vi "Module - Page Master Data.vi"(11 "Stop":bool) -> ()   [LabVIEW 2020]
uses:
  Control/Setup - Sequence Data.ctl
  Control/State - eFGV.ctl
panel:
  in  "Tab Control":enum32{"Test Procedure", "Layout"}(tab)
  in  "Header multi-test":T1={"Test Type"="Test Requirement", "Seq.Done"="Done", "Seq.No"="No.", "Seq.SelectRun"="Run", "Seq.SelectRun 2"="Test Sequence", "Seq.SelectRun 3"="Test Requirement ID", "Test Type 2"="Test Procedure", "Test Type 3"="psi", "Test Type 4"="Test Pressure", "Test Type 5"="Secondary", "Test Type 6"="Tertiary", "Test Type 7"="Primary", "Test Type 8"="Holding Time (hh:mm)", "Test Type 9"="Section", "Test Type 10"="Test Media", "Test Type 11"="psi", "Test Type 12"="Actuator Pressure", "Test Type 13"="psi/hour", "Test Type 14"="Chart scale", "Test Type 15"="2nd", "Test Type 16"="3rd", "Test Type 17"="1st", "Test Type 18"="Blowdown", "Test Type 19"="psi", "Test Type 20"="Max. Blowdown Pressure", "Seq.SelectRun 4"=""}
  in  "SequenceList":T2[](array[typedef])
  out "Procedure Details Label":string="Procedure Details" caption="Procedure Details"
  out "Indicator.PSL":string caption="PSL"
  out "Indicator.Rev.":string caption="Rev."
  out "Indicator.Procedure No./Ref.":string caption="Procedure No./Ref."
  in  "Procedure Detail.Save":bool
  in  "Button.Edit.Test Procedure.":bool caption="Edit"
  in  "Button.New.Test Procedure":bool caption="New"
  in  "Button.Test Procedure.Copy":bool caption="Copy"
  in  "Button.Search.Test Procedure":bool caption="Search"
  in  "PSL.Control":string(combo) caption="PSL"
  in  "Rev.Control":string caption="Rev."
  in  "Procedure No./Ref.Control":string caption="Procedure No./Ref."
  out "Test Procedure.Selection Label":string="Selection" caption="Selection Label"
  out "Test Procedure Label":string="Test Procedure"
  out "Control.Layout Technical Name":string caption="Layout Technical Name"
  in  "Checkbox.Output":bool caption="Output"
  in  "Checkbox.Default":bool caption="Default"
  in  "Control.Layout Name":string caption="Layout Name"
  in  "Conntrol.Layout ID":u16 caption="Layout ID"
  out "Indicator.Output Name":string caption="Output Name"
  in  "Listbox.Output Type":string(combo) caption="Output Type"
  in  "Control.Company Name":string caption="Company Name"
  out "Indicator.Output Set":u16 caption="Output Set"
  out "Ouput.Layout Detail Label":string="Layout Detail"
  in  "Button.Output.Search":bool caption="Search"
  in  "Button.Edit.Output":bool caption="Edit"
  in  "Button.New.Output":bool caption="New"
  in  "Button.Output.Copy":bool caption="Copy"
  out "Company Name.Indicator":string
  out "Ouput.Selection Label":string="Selection"
  in  "Control.Output Set":u16 caption="Output Set"
  out "Output Label":string="Output"
  # "MASTER DATA"
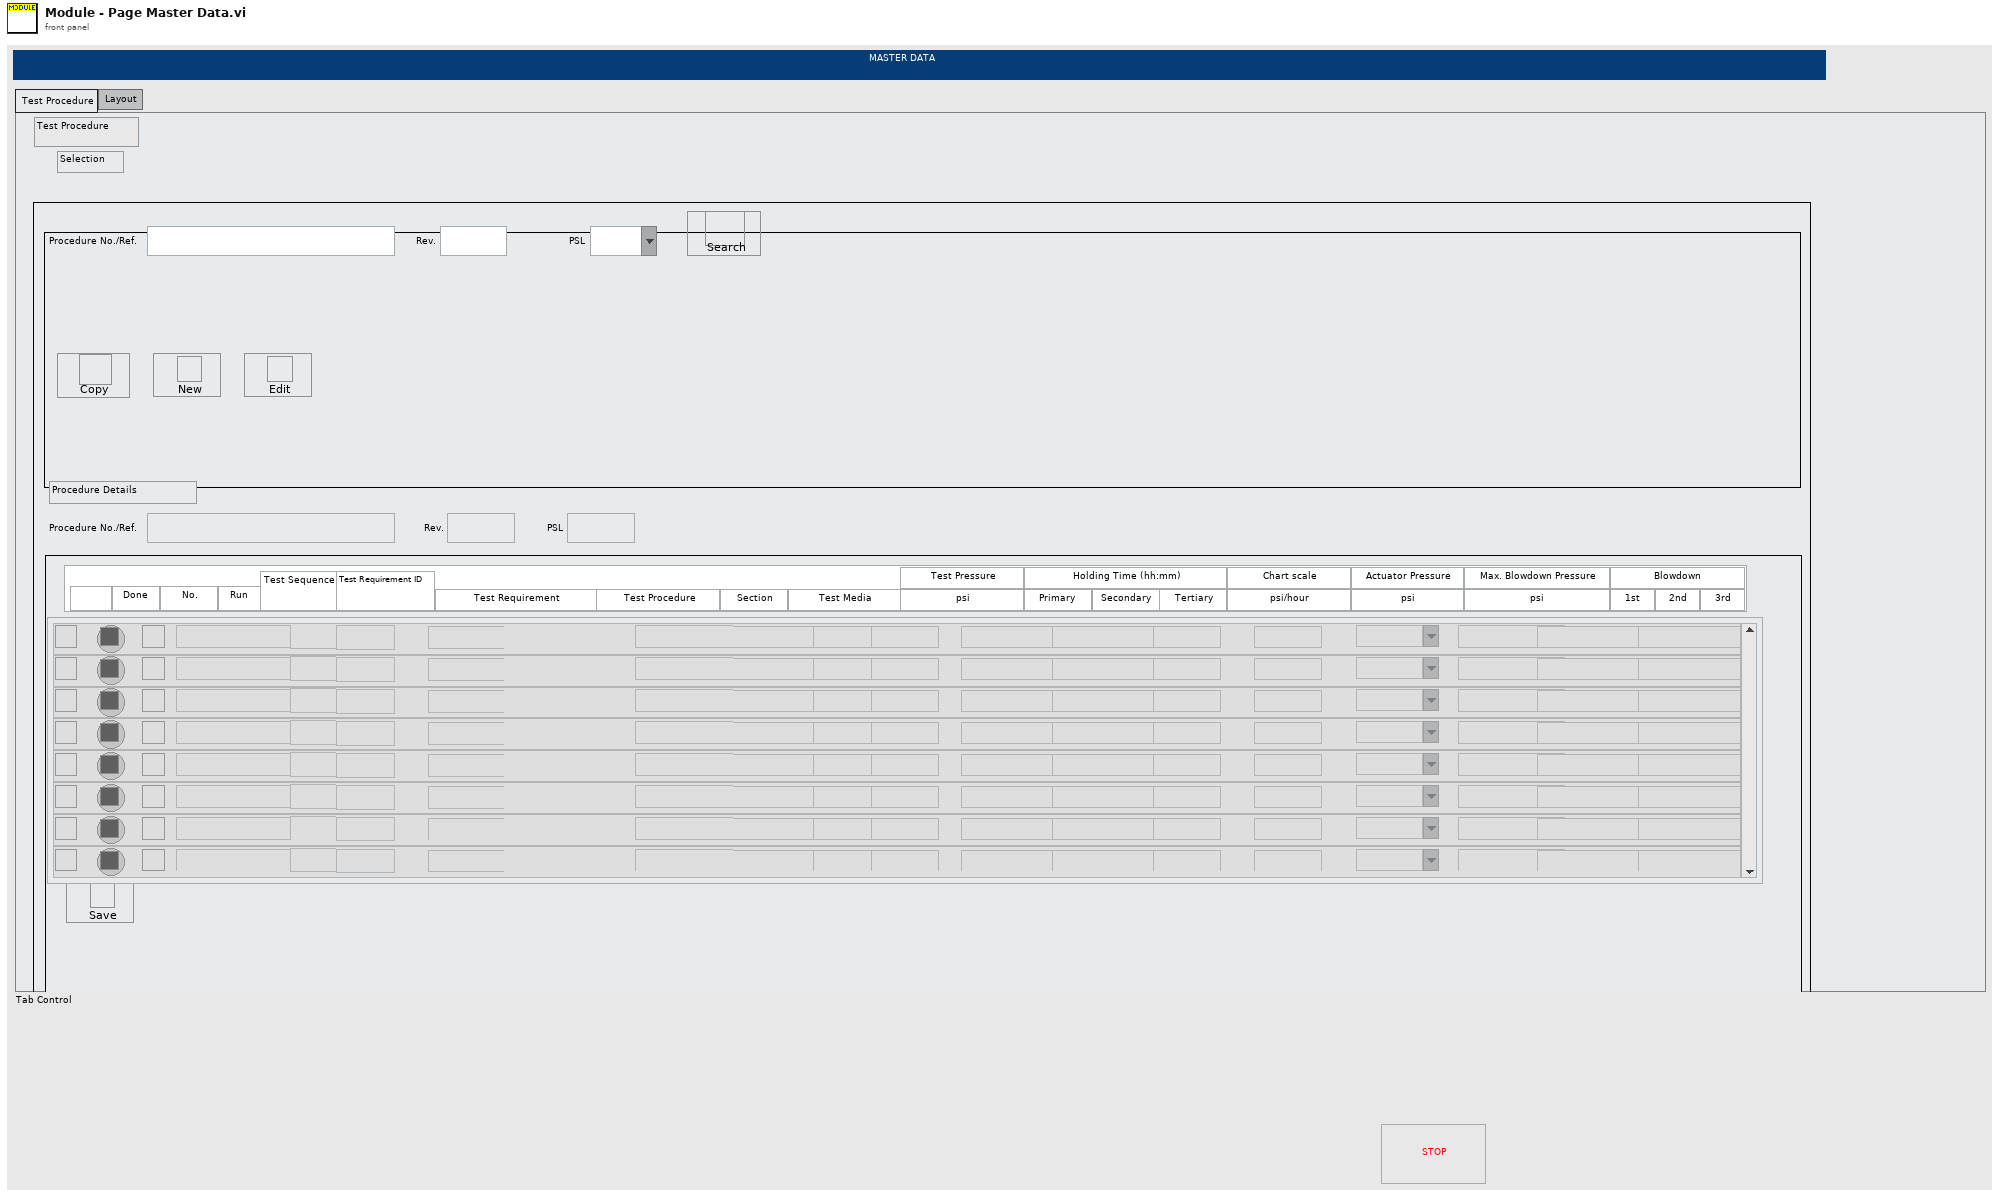
[diagram p1: front panel]
types:
  T1 = cluster{"Test Type":string, "Seq.Done":string, "Seq.No":string, "Seq.SelectRun":string, "Seq.SelectRun 2":string, "Seq.SelectRun 3":string, "Test Type 2":string, "Test Type 3":string, "Test Type 4":string, "Test Type 5":string, "Test Type 6":string, "Test Type 7":string, "Test Type 8":string, "Test Type 9":string, "Test Type 10":string, "Test Type 11":string, "Test Type 12":string, "Test Type 13":string, "Test Type 14":string, "Test Type 15":string, "Test Type 16":string, "Test Type 17":string, "Test Type 18":string, "Test Type 19":string, "Test Type 20":string, "Seq.SelectRun 4":string}
  T2 = typedef "Setup - Sequence Data.ctl" = cluster{"Seq.Select":bool, "Seq.Status":u32, "Seq.Run":bool, "Seq.TestSequence":string, "Seq.No":string, "Seq.ReqID":string, "Seq.TestReq":string, "Seq.Variance":string, "Seq.TestProcedure":string, "Seq.Section":string, "Seq.TestBunker":string, "Seq.TestMedia":string, "Seq.TestPressure":string, "Seq.Cycle":string, "Seq.HoldingTime":string, "Seq.ChartScale":string, "Seq.BDIndicator":string, "Seq.ActuatorPressure":string, "Seq.MaxBDPressure":string}
  T3 = cluster{"T_Out":i32, "Event Ref":refnum<event-registration>}
  T4 = enum16{"Init", "Register Event", "Idle", "Process", "Close"}
  T5 = typedef "State - eFGV.ctl" = enum16{"Init", "Read", "Write", "Exit"}
  T6 = enum32{"invalid app kind", "Development System", "Run Time System", "Student Edition", "Embedded LabVIEW", "Evaluation", "Custom"}
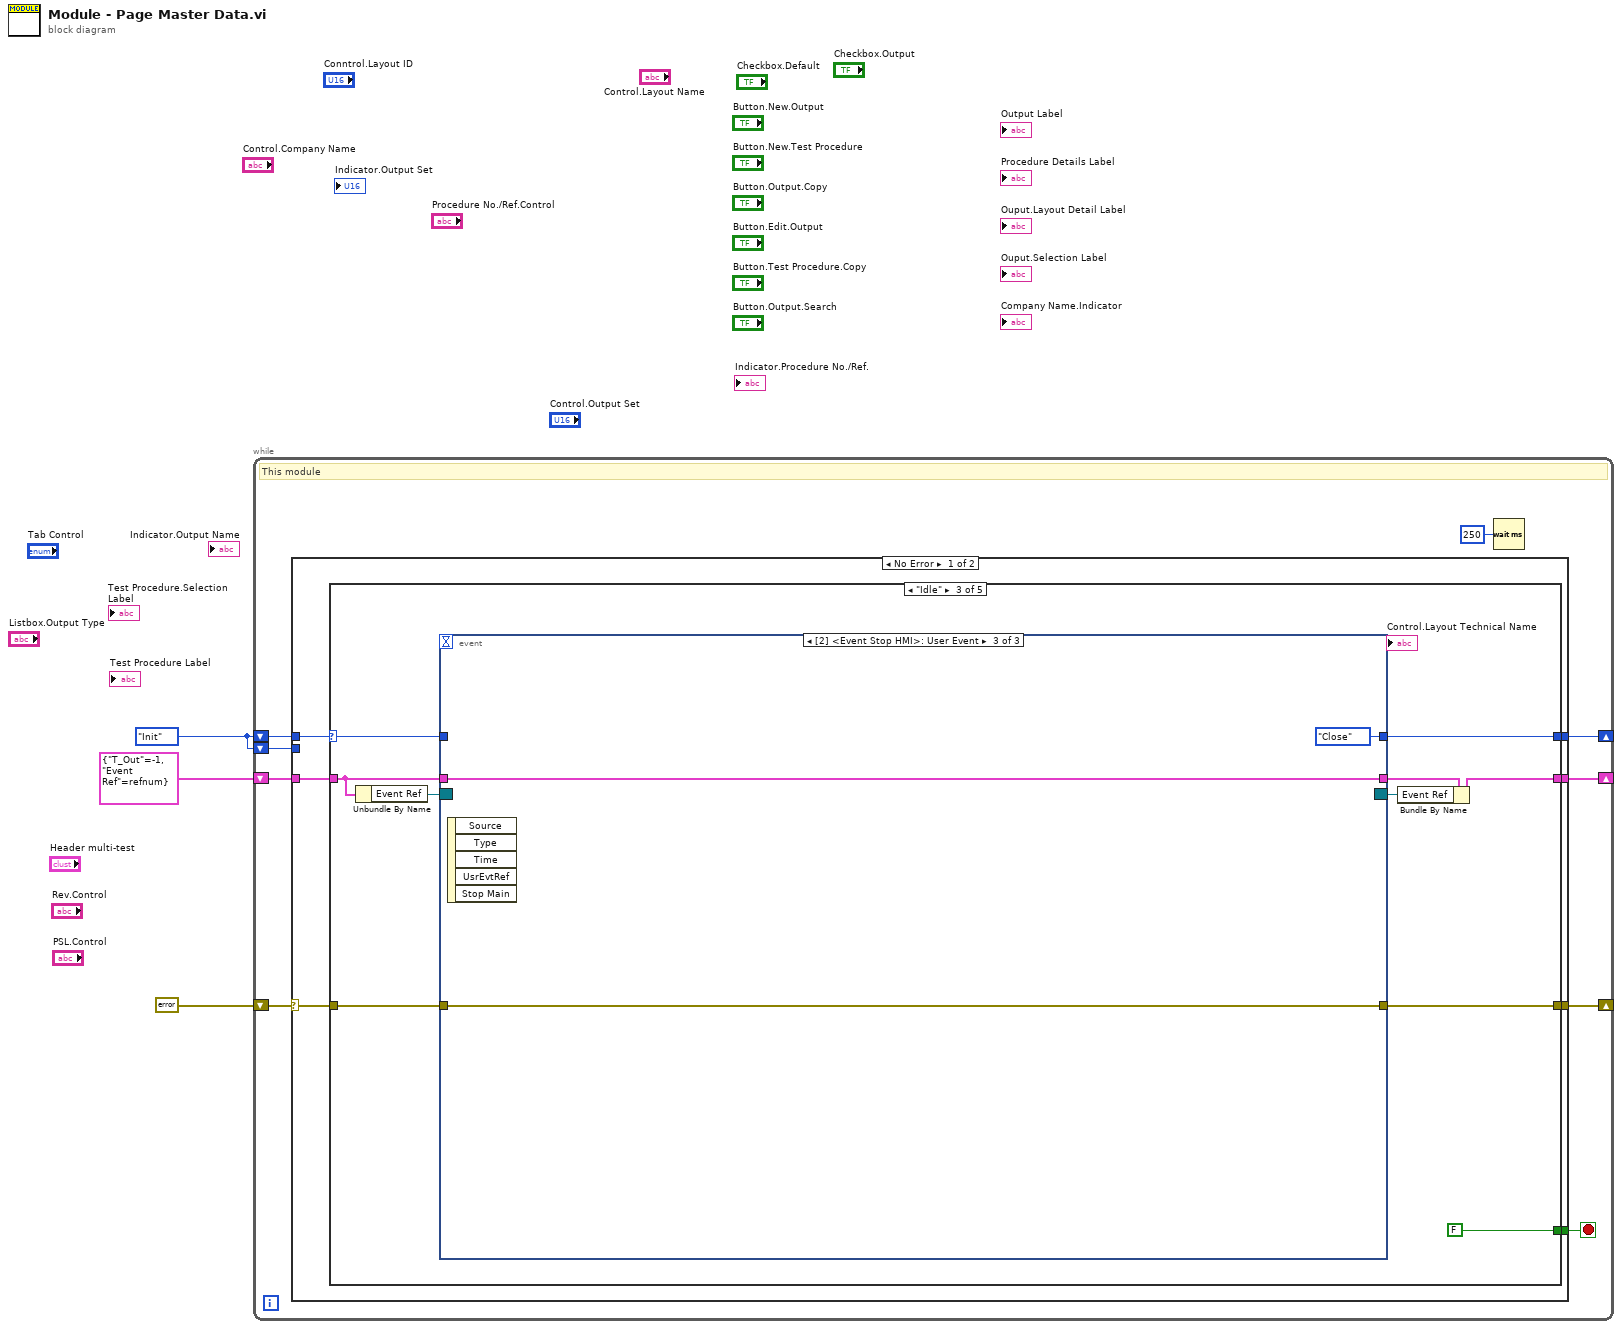
[diagram p0: block diagram]
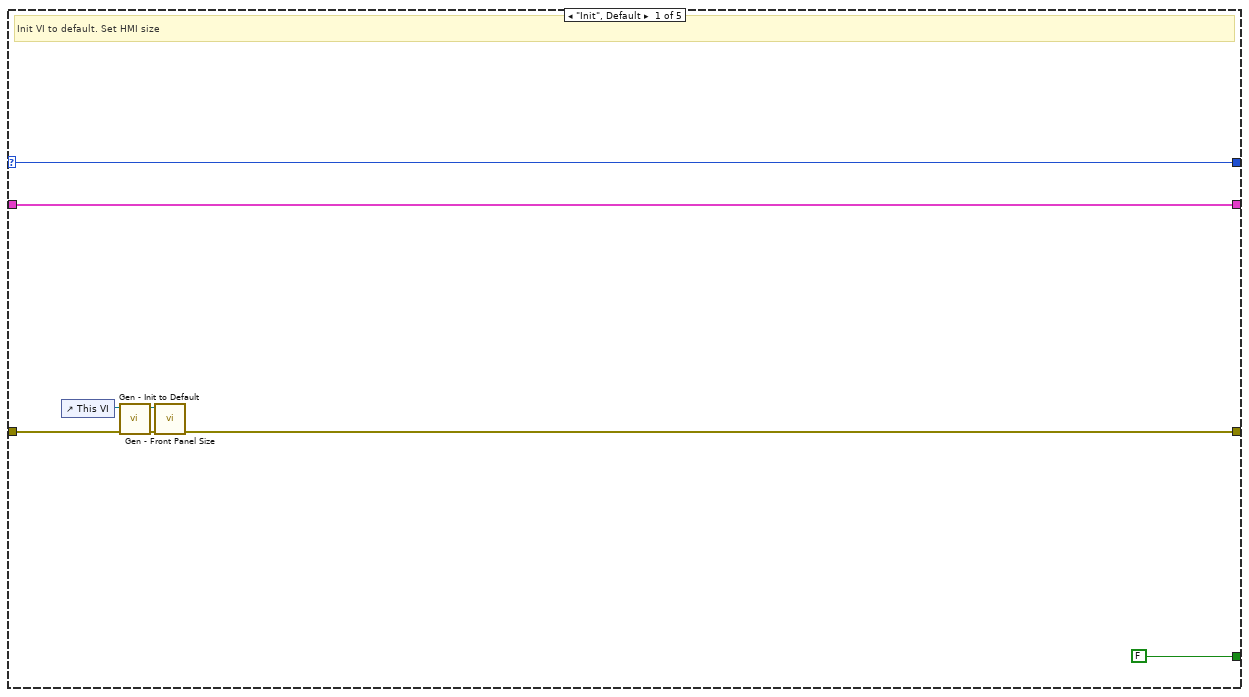
[diagram p2: hidden frame]
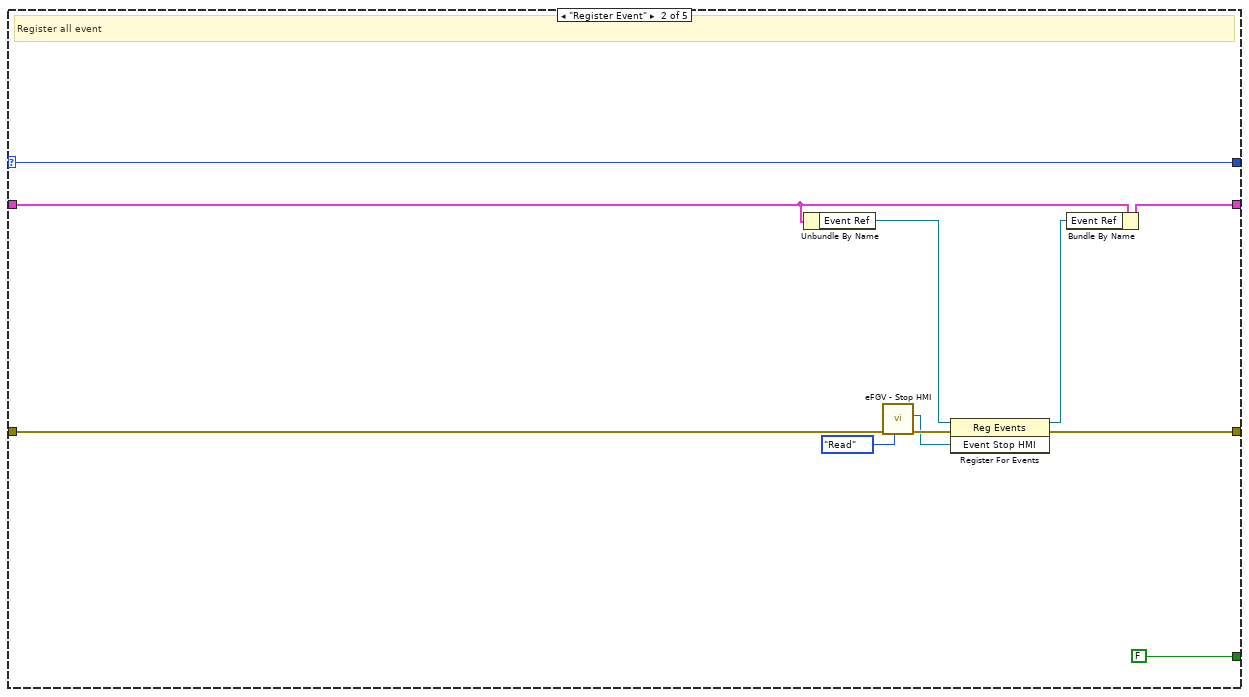
[diagram p3: hidden frame]
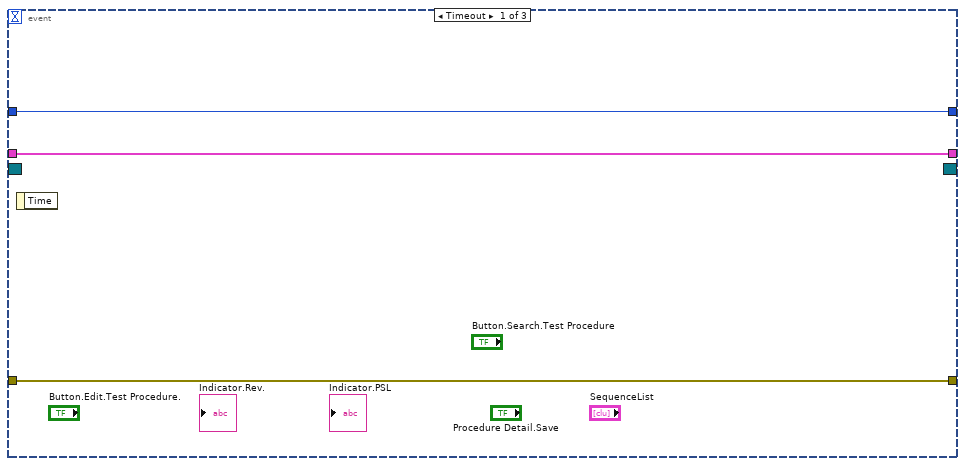
[diagram p4: hidden frame]
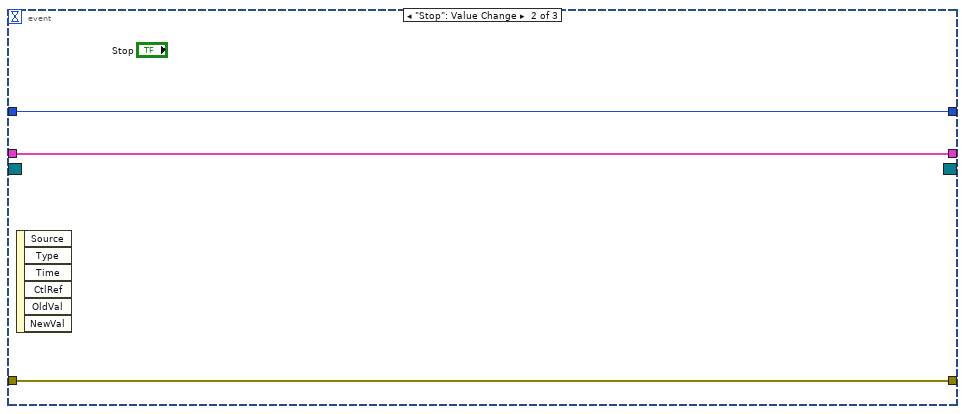
[diagram p5: hidden frame]
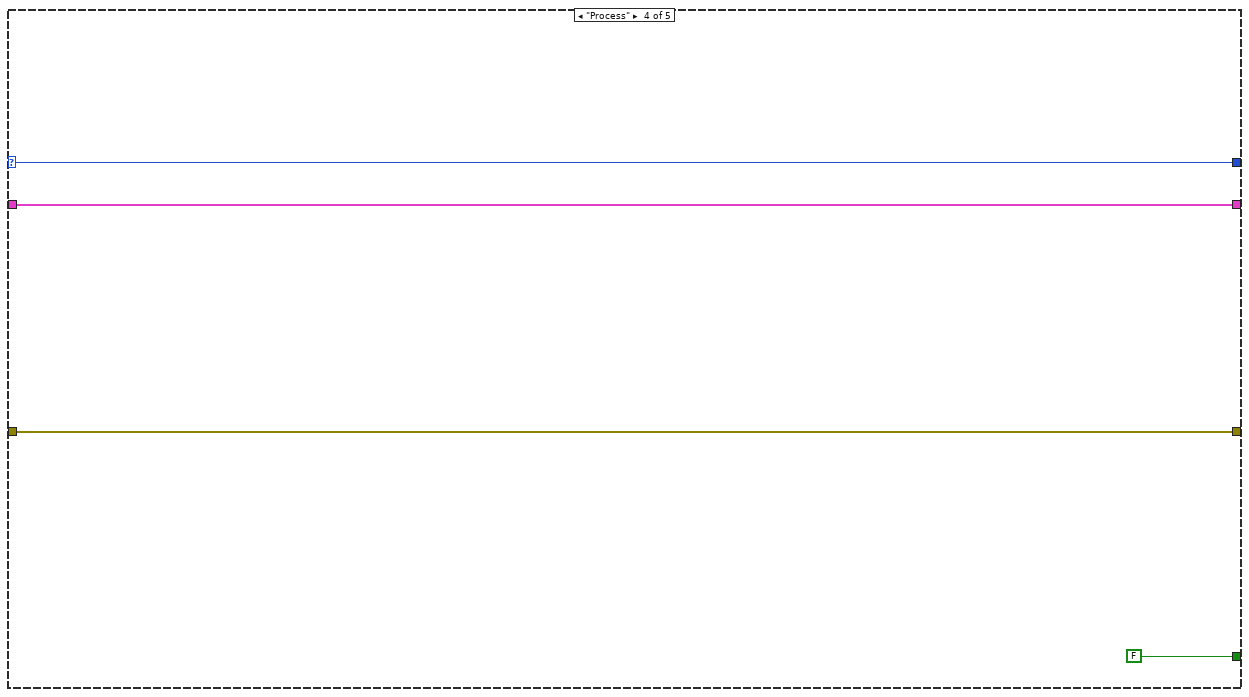
[diagram p6: hidden frame]
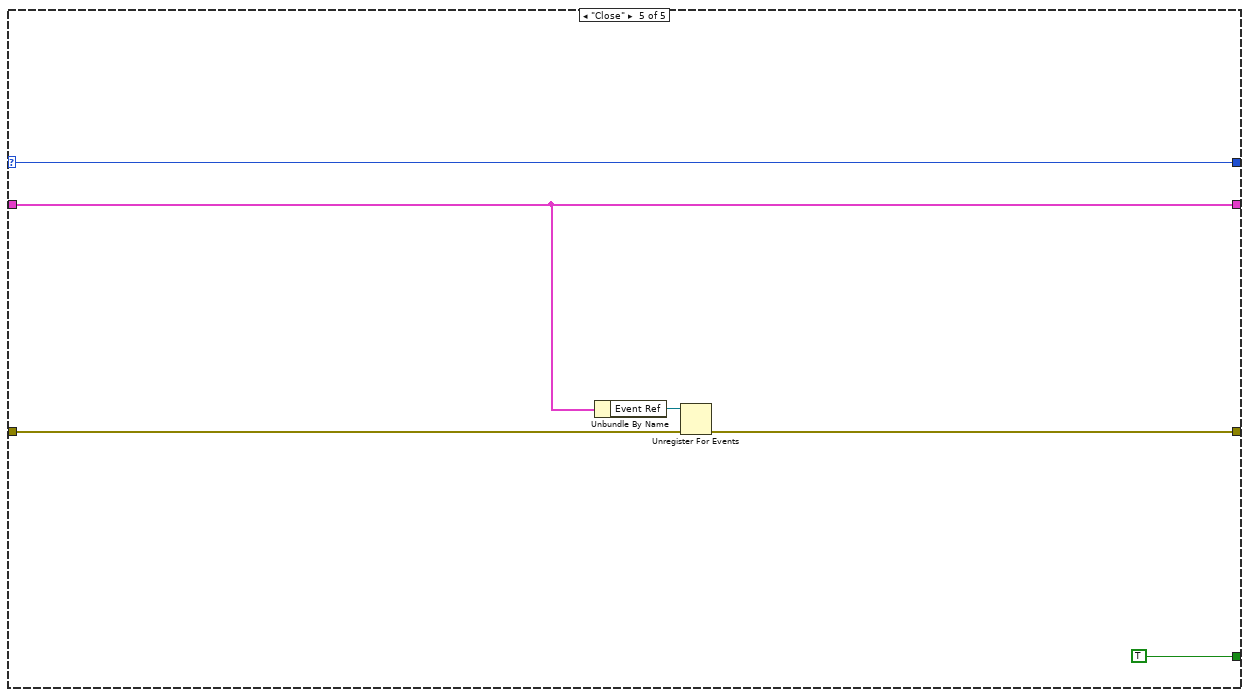
[diagram p7: hidden frame]
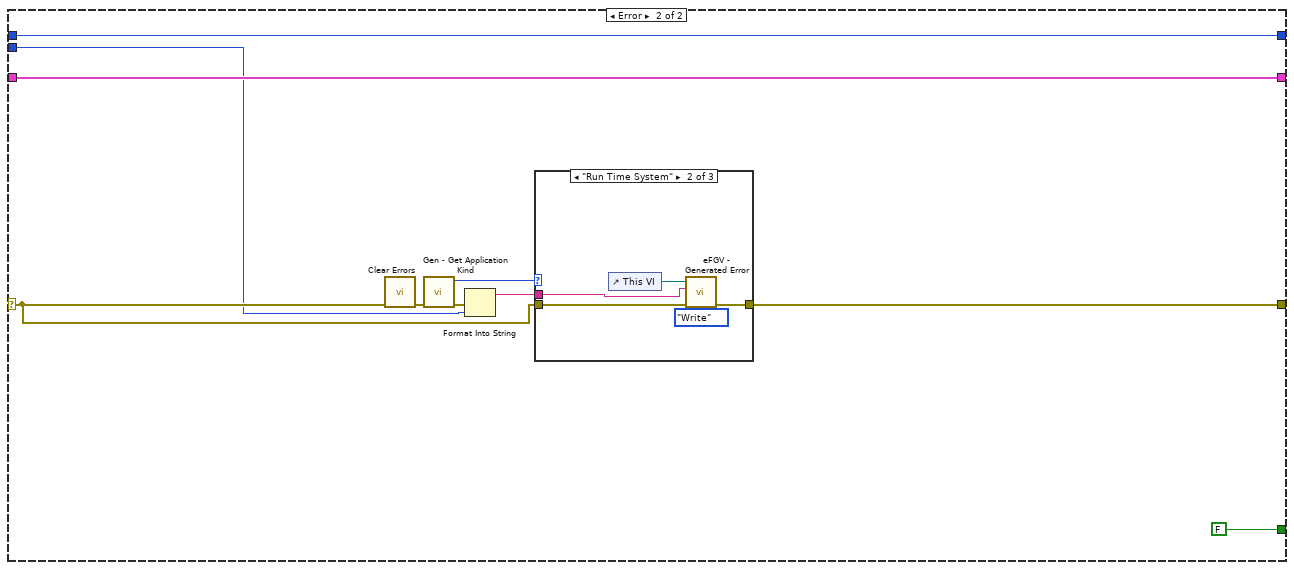
[diagram p8: hidden frame]
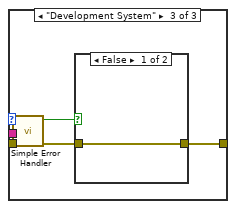
[diagram p10: hidden frame]
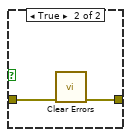
[diagram p11: hidden frame]
diagram:
  w1 = T4."Init"
  n1 = while {
    shift-right: [w8] -> _
    shift-left: w1 -> [w10]
    shift-right: [w11] -> _
    shift-left: errorcluster {"status"=FALSE, "code"=0, "source"=""} ("Error In") -> [w12]
    shift-right: [w6] -> _
    shift-left: T3 {"T_Out"=-1, "Event Ref"=refnum} -> [w7]
    shift-left: w1 -> [w4]
    stop <- w9 stop-if-true
    # "This module"
    n2 = case shown="No Error" w12 {
      selector: w12 -> [w18 w71]
      tunnel: w10 -> [w17 w76]
      tunnel: [w19 w72] -> w11
      tunnel: [w16 FALSE] -> w9
      tunnel: [w15 w76] -> w8
      tunnel: w7 -> [w14 w75]
      tunnel: [w13 w75] -> w6
      tunnel: w4 -> [_ w68]
      frame No Error {
        n3 = case shown="\"Idle\"" w17 {
          selector: w17 -> [w22 w34 w43 w58 w65]
          tunnel: [w25 w38 w48 w61 w66] -> w19
          tunnel: w18 -> [w27 w36 w47 w61 w67]
          tunnel: [FALSE FALSE FALSE FALSE TRUE] -> w16
          tunnel: [w22 w34 w45 w58 w65] -> w15
          tunnel: w14 -> [w24 w31 w42 w59 w63]
          tunnel: [w24 w29 w40 w59 w63] -> w13
          frame "Init", Default {
            # "Init VI to default. Set HMI size"
            n4 = control-ref of="This VI"() -> (w21:refnum<vi>)
            n5 = call "Gen - Init to Default.vi"("Error in"=w27, "This VI"=w21) -> ("Error out"=w26:errorcluster, "This VI Copy"=w20:refnum<vi>)  [unwired: 8 in]
            n6 = call "Gen - Front Panel Size.vi"("Error In"=w26, "This VI"=w20) -> ("Error Out"=w25:errorcluster)  [unwired: 9 in]
          }
          frame "Register Event" {
            # "Register all event"
            n7 = Unbundle By Name(w31) -> ("Event Ref"=w30:refnum<event-registration>)
            n8 = call "eFGV - Stop HMI.vi"("Action"=State_-_eFGV."Read", "Error In"=w36) -> ("Error Out"=w37:errorcluster, "Event Stop HMI"=w33:refnum<user-event>)  [unwired: 7 in, 1 out]
            n9 = register-events(reference=w30, error in=w37, w33) -> (reference out=w28:refnum<event-registration>, error out=w38:errorcluster)
            n10 = Bundle By Name(cluster=w31, "Event Ref"=w28) -> (w29:T3)
          }
          frame "Idle" {
            n11 = Unbundle By Name(w42) -> ("Event Ref"=w41:refnum<event-registration>)
            n12 = event shown="[2] <Event Stop HMI>: User Event" {
              selector: w41 -> [_ _ _]
              dyn-events: [_ _ _] -> w39
              timeout: _ -> [_ _ _]
              tunnel: [w51 w54 w57] -> w48
              tunnel: w47 -> [w51 w54 w57]
              tunnel: [w49 w52 T4."Close"] -> w45
              tunnel: [w50 w53 w56] -> w44
              tunnel: w42 -> [w50 w53 w56]
              tunnel: w43 -> [w49 w52 _]
              event Timeout {
                n13 = event-data() -> ()  [unwired: 1 in, 1 out]
              }
              event "Stop": Value Change {
                n14 = event-data() -> ()  [unwired: 1 in, 6 out]
              }
              event User Event {
                n15 = event-data() -> ()  [unwired: 1 in, 5 out]
              }
            }
            n16 = Bundle By Name(cluster=w44, "Event Ref"=w39) -> (w40:T3)
          }
          frame "Process" {
          }
          frame "Close" {
            n17 = Unbundle By Name(w63) -> ("Event Ref"=w62:refnum<event-registration>)
            n18 = Unregister For Events(event registration refnum=w62, error in=w67) -> (error out=w66:errorcluster)
          }
        }
      }
      frame Error {
        n19 = call <vilib>:"Clear Errors.vi"("error in (no error)"=w71) -> ("error out"=w74:errorcluster)  [unwired: 5 in, 1 out]
        n20 = call "Gen - Get Application Kind.vi"("Error In"=w74) -> ("Error Out"=w70:errorcluster, "Application:Kind"=w73:T6)  [unwired: 9 in]
        n21 = Format Into String(error in=w70, w68) -> (resulting string=w69:string)  [unwired: 2 in, 1 out]
        n22 = case shown="\"Run Time System\"" w73 {
          tunnel: [w78 w83 w87] -> w72
          tunnel: w71 -> [w78 w80 w85]
          tunnel: w69 -> [_ w79 _]
          frame "invalid app kind", Default {
          }
          frame "Run Time System" {
            n23 = control-ref of="This VI"() -> (w81:refnum<vi>)
            n24 = call "eFGV - Generated Error.vi"("eFGV States"=State_-_eFGV."Write", "Error In"=w80, "State"=w79, "This VI"=w81) -> ("Error Out"=w83:errorcluster)  [unwired: 6 in, 1 out]
          }
          frame "Development System" {
            n25 = call <vilib>:"Simple Error Handler.vi"("error in (no error)"=w85) -> ("error?"=w84:bool, "error out"=w86:errorcluster)  [unwired: 4 in, 3 out]
            n26 = case shown="False" w84 {
              tunnel: [w88 w90] -> w87
              tunnel: w86 -> [w88 w89]
              frame False {
              }
              frame True {
                n27 = call <vilib>:"Clear Errors.vi"("error in (no error)"=w89) -> ("error out"=w90:errorcluster)  [unwired: 5 in, 1 out]
              }
            }
          }
        }
      }
    }
    n28 = Wait (ms)(milliseconds to wait=u32 250) -> ()  [unwired: 1 out]
  }
